vi "build auth URI.vi"(8 "error in (no error)":errorcluster, 10 "State Parameter":string, 11 "Oauth2 in":refnum<class "Oauth2.lvclass">) -> (0 "error out":errorcluster, 2 "Authorization Request URI":string, 3 "Oauth2":refnum<class "Oauth2.lvclass">)   [LabVIEW 2020, in "Oauth2.lvclass"]
uses:
  Oauth2.lvclass
  Oauth2.lvclass/Oauth2.ctl
  <vilib>/LabVIEW Open Source Project/OpenSerializer.Base64/Serializer.Base64.lvclass/Serializer.Base64.ctl
  <vilib>/LabVIEW Open Source Project/OpenSerializer.Base64/Serializer.Base64.lvclass
  <vilib>/LabVIEW Open Source Project/OpenURI/uri/URI.lvclass
  <vilib>/LabVIEW Open Source Project/Unicity/RandomStringGenerator/RandomStringGenerator.lvclass
  OAuthToken/OAuth2 Token Element -- enum.ctl
  OAuthToken/OAuthAccessToken.lvclass
  <vilib>/LabVIEW Open Source Project/OpenURI/openURI.lvlib
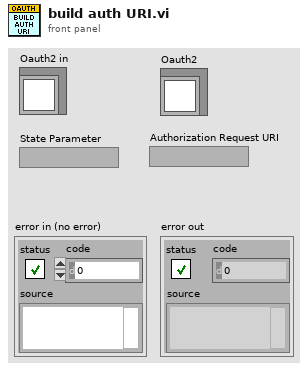
[diagram p1: front panel]
types:
  T1 = typedef "OAuthAccessToken.lvclass/OAuth2 Token Element -- enum.ctl" = enum16{"client_id", "client_secret", "response_type", "scope", "redirect_uri", "error", "error_description", "error_uri", "grant_type", "code", "access_token", "token_type", "expires_in", "username", "password", "refresh_token", "code_challenge", "code_challenge_method", "reverse_proxy_uri", "endpoint element"}
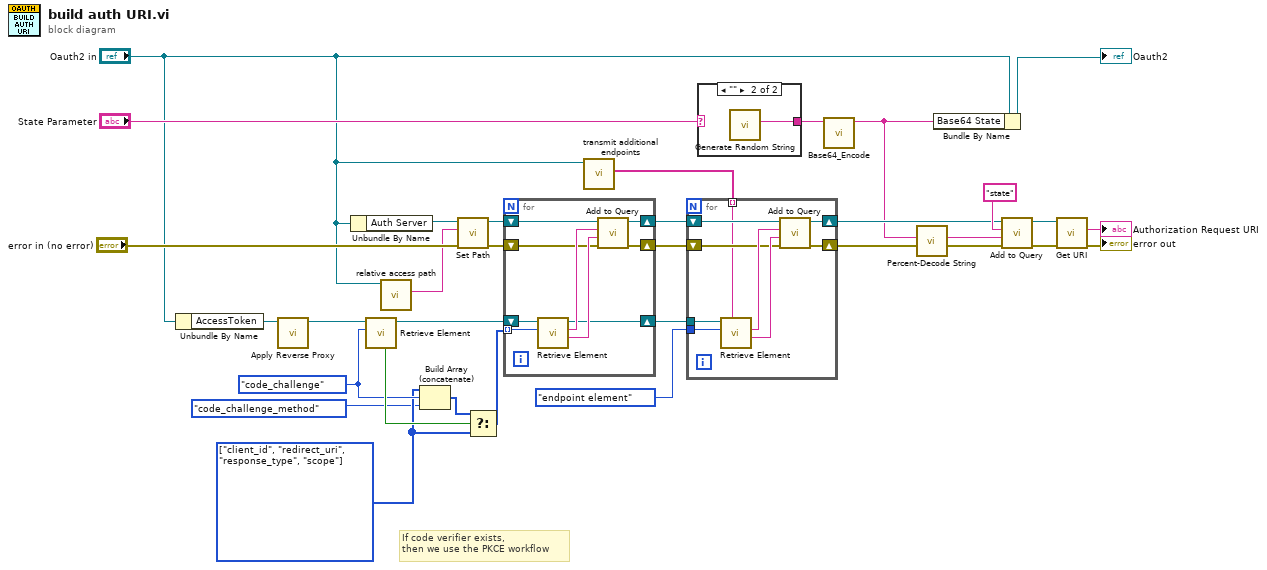
[diagram p0: block diagram]
diagram:
  w11 = OAuth2_Token_Element_--_enum."code_challenge" ("Token element")
  w9 = T1[] [enum."client_id", enum."redirect_uri", enum."response_type", enum."scope"] items=["client_id", "client_secret", "response_type", "scope", "redirect_uri", "error", "error_description", "error_uri", "grant_type", "code", "access_token", "token_type", "expires_in", "username", "password", "refresh_token", "code_challenge", "code_challenge_method", "reverse_proxy_uri", "endpoint element"]
  # "If code verifier exists, \nthen we use the PKCE workflow"
  n1 = Unbundle By Name("Oauth2 in") -> ("AccessToken"=w2:refnum<class "OAuthAccessToken.lvclass">)
  n2 = call "Apply Reverse Proxy.vi"("OAuthAccessToken in"=w2) -> ("OAuthAccessToken out"=w1:refnum<class "OAuthAccessToken.lvclass">)  [unwired: 9 in, 1 out]
  n3 = Unbundle By Name("Oauth2 in") -> ("Auth Server"=w29:refnum<class "URI.lvclass">)
  n4 = call "Retrieve Element.vi"("Token element"=w11, "OAuthAccessToken in"=w1) -> ("OAuthAccessToken out"=w13:refnum<class "OAuthAccessToken.lvclass">, "element found"=w12:bool)  [unwired: 5 in, 3 out]
  n5 = call-dynamic "relative access path.vi"("Oauth2 in"="Oauth2 in") -> ("Authorization Path"=w27:string)  [unwired: 9 in, 1 out]
  n6 = Build Array (concatenate)(w9, w11, OAuth2_Token_Element_--_enum."code_challenge_method" ("Token element")) -> (w10:T1[])
  n7 = call <vilib>:"Set Path.vi"("error in (no error)"="error in (no error)", "path"=w27, "URI in"=w29) -> ("error out"=w23:errorcluster, "URI out"=w24:refnum<class "URI.lvclass">)  [unwired: 7 in]
  n8 = Select(t=w10, s=w12, f=w9) -> (s? t:f=w8:T1[])
  n9 = for {
    tunnel: w8 -> [w40] mode=indexing
    shift-right: [w38] -> w22
    shift-left: w24 -> [w39]
    shift-right: [w34] -> w20
    shift-left: w23 -> [w35]
    shift-right: [w33] -> w17
    shift-left: w13 -> [w41]
    n10 = call "Retrieve Element.vi"("Token element"=w40, "OAuthAccessToken in"=w41) -> ("Value"=w36:string, "Key"=w37:string, "OAuthAccessToken out"=w33:refnum<class "OAuthAccessToken.lvclass">)  [unwired: 5 in, 2 out]
    n11 = call <vilib>:"Add to Query.vi"("error in (no error)"=w35, "value"=w36, "key"=w37, "URI in"=w39) -> ("error out"=w34:errorcluster, "URI out"=w38:refnum<class "URI.lvclass">)  [unwired: 6 in]
  }
  n12 = call-dynamic "transmit additional endpoints.vi"("Oauth2"="Oauth2 in") -> ("Additional Endpoints"=w18:string[])  [unwired: 10 in]
  n13 = for {
    tunnel: w17 -> [w50]
    shift-right: [w48] -> w21
    shift-left: w22 -> [w49]
    shift-right: [w44] -> w19
    shift-left: w20 -> [w45]
    tunnel: w18 -> [w42] mode=indexing
    tunnel: OAuth2_Token_Element_--_enum."endpoint element" ("Token element") -> [w43]
    n14 = call "Retrieve Element.vi"("Endpoint element key"=w42, "Token element"=w43, "OAuthAccessToken in"=w50) -> ("Value"=w46:string, "Key"=w47:string)  [unwired: 4 in, 3 out]
    n15 = call <vilib>:"Add to Query.vi"("error in (no error)"=w45, "value"=w46, "key"=w47, "URI in"=w49) -> ("error out"=w44:errorcluster, "URI out"=w48:refnum<class "URI.lvclass">)  [unwired: 6 in]
  }
  n16 = case shown="\"\"" "State Parameter" {
    selector: "State Parameter" -> [w51 _]
    tunnel: [w51 w52] -> w26
    frame Default {
    }
    frame "" {
      n17 = call <vilib>:"Generate Random String.vi"() -> ("Random String"=w52:string)  [unwired: 11 in]
    }
  }
  n18 = call <vilib>:"Base64_Encode.vi"("String"=w26) -> ("Encoded String"=w15:string)  [unwired: 9 in, 1 out]
  n19 = call <vilib>:"Percent-Decode String.vi"("Pct-Encoded String"=w15) -> ("String"=w14:string)  [unwired: 10 in]
  n20 = Bundle By Name(cluster="Oauth2 in", "Base64 State"=w15) -> (→"Oauth2":refnum<class "Oauth2.lvclass">)
  n21 = call <vilib>:"Add to Query.vi"("error in (no error)"=w19, "value"=w14, "key"="state" ("argument"), "URI in"=w21) -> ("error out"=w4:errorcluster, "URI out"=w5:refnum<class "URI.lvclass">)  [unwired: 6 in]
  n22 = call <vilib>:"Get URI.vi"("error in (no error)"=w4, "URI in"=w5) -> ("error out"=→"error out":errorcluster, "URI String"=→"Authorization Request URI":string)  [unwired: 7 in, 1 out]
